vi "start daemon.vi"(8 "error in (no error)":errorcluster) -> (0 "error out":errorcluster)   [LabVIEW 2016, in "update.lvlib"]
uses:
  update.lvlib
panel:
  out "standard error":string caption="标准错误"
  out "standard output":string caption="标准输出"
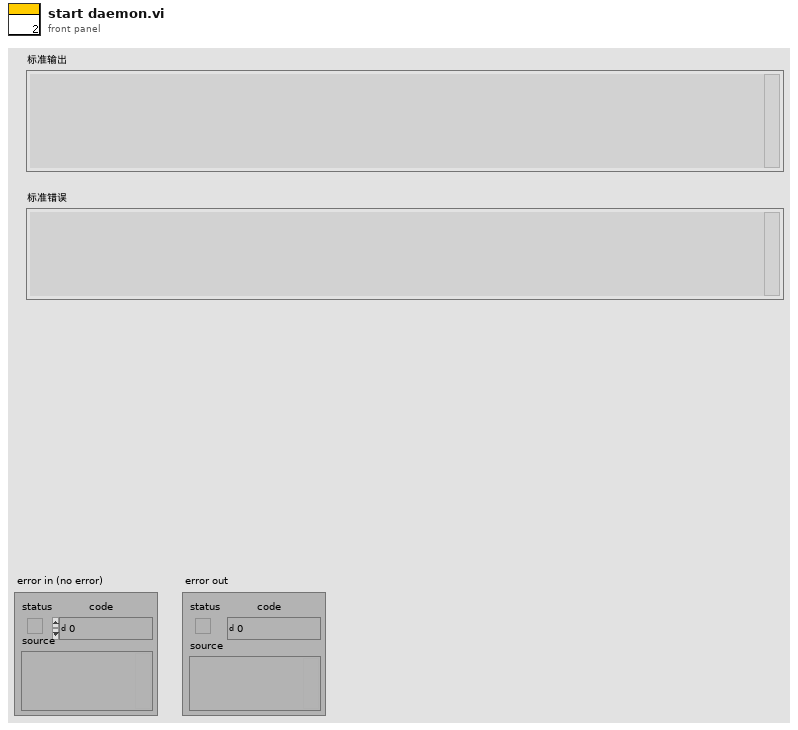
[diagram p1: front panel]
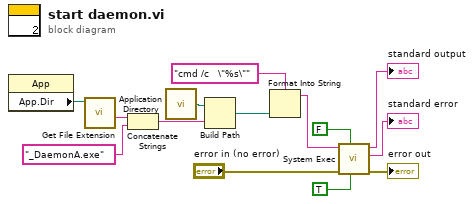
[diagram p0: block diagram]
diagram:
  n1 = property class="App"() -> ("App.Dir"=w12:path)  [unwired: 2 in, 2 out]
  n2 = call <vilib>:"Get File Extension.vi"("file"=w12) -> ("filename without extension"=w11:string)  [unwired: 6 in, 4 out]
  n3 = Concatenate Strings(w11, "_DaemonA.exe" ("名称或相对路径")) -> (w3:string)
  n4 = call <vilib>:"Application Directory.vi"() -> ("Application Directory"=w4:path)
  n5 = Build Path(base path=w4, name or relative path=w3) -> (appended path=w1:path)
  n6 = Format Into String(format string="cmd /c   \"%s\"" ("格式字符串"), w1) -> (resulting string=w10:string)  [unwired: 2 in, 1 out]
  n7 = call <vilib>:"System Exec.vi"("run minimized? (F)"=TRUE, "wait until completion? (T)"=FALSE, "error in (no error)"="error in (no error)", "command line"=w10) -> ("error out"=→"error out":errorcluster, "standard error"=→"standard error":string, "standard output"=→"standard output":string)  [unwired: 4 in, 1 out]
